vi "Skips the selected step for AUTO.vi"(8 "error in":errorcluster, 9 "Setup the Skip Step Status":u8(ring) items=["OFF", "ON"], 10 "Select Step for Skip":u8=1 min=1 max=16, 11 "VISA resource name":refnum<visa-resource-name>) -> (0 "error out":errorcluster, 3 "VISA resource name out":refnum<visa-resource-name>)   [LabVIEW 2011, in "GPT-9000.lvlib"]
uses:
  <instrlib>/GPT-9000/GPT-9000.lvlib
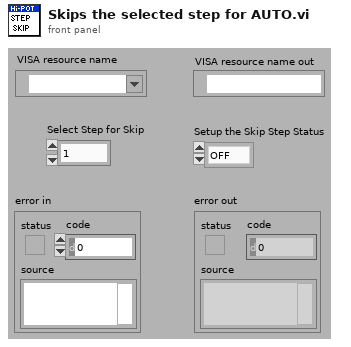
[diagram p1: front panel]
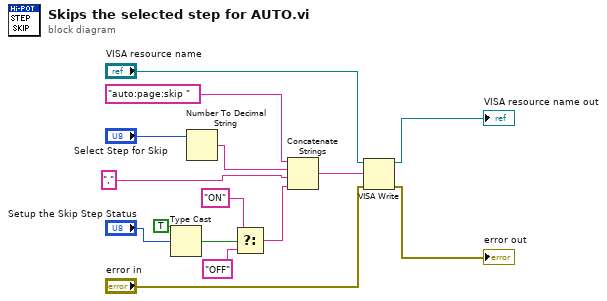
[diagram p0: block diagram]
diagram:
  n1 = Type Cast(type=TRUE, x="Setup the Skip Step Status") -> (*(type *) &x=w4:bool)
  n2 = Number To Decimal String(number="Select Step for Skip") -> (decimal integer string=w13:string)  [unwired: 1 in]
  n3 = Select(t="ON", s=w4, f="OFF") -> (s? t:f=w1:string)
  n4 = Concatenate Strings("auto:page:skip ", w13, ",", w1) -> (w9:string)
  n5 = VISA Write(VISA resource name="VISA resource name", write buffer=w9, error in (no error)="error in") -> (VISA resource name out=→"VISA resource name out":refnum<visa-resource-name>, error out=→"error out":errorcluster)  [unwired: 1 out]
